vi "I32 to Data Type.vi"(8 "error in (no error)":errorcluster, 11 "I32":i32) -> (0 "error out":errorcluster, 3 "Boolean out":refnum<class "I32.lvclass">)   [LabVIEW 2020, in "I32.lvclass"]
uses:
  <vilib>/gpm_packages/@cs/data-type-serializer/source/I32/I32.lvclass
  <vilib>/gpm_packages/@cs/data-type-serializer/source/I32/I32.lvclass/I32.ctl
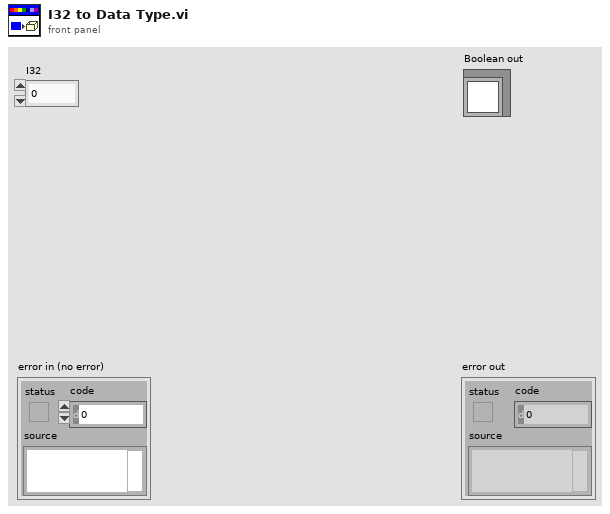
[diagram p1: front panel]
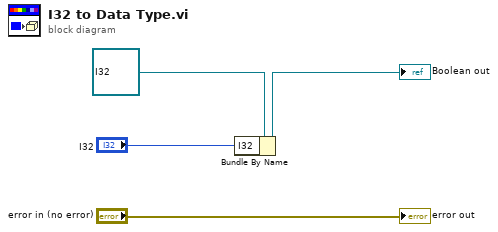
[diagram p0: block diagram]
diagram:
  n1 = Bundle By Name(cluster=refnum<class "I32.lvclass"> refnum ("Boolean in"), "I32"="I32") -> (→"Boolean out":refnum<class "I32.lvclass">)
  "error out" <- "error in (no error)"
